vi "esp8266_test1.3.vi"() -> ()   [LabVIEW 2012]
doc: "1.2.2\n加入手动破解无线功能\n1.2.3\n由手动改为半自动破解\n1.2.4\n全自动破解与半自动破解并存模式"
uses:
  <vilib>/Instr/_visa.llb/VISA Configure Serial Port (Instr).vi
panel:
  out "String":string
  out "正常":bool
  out "透传":bool
  in  "停止":bool
  out "错误输出 2":errorcluster caption="错误输出"
  in  "清空":bool
  in  "?":enum32{"配置", "选网", "远程", "接口", "关于"}(tab)
  in  "VISA":refnum<visa-resource-name> caption="VISA资源名称"
  in  "baud rate (9600)":u32=9600
  in  "data bits (8)":u16=8 min=5 max=8 step=1
  in  "修改波特率":bool
  in  "组合框":string(combo)
  in  "模式设置":bool
  in  "模式":u32(ring) items=["无", "station模式", "AP模式", "双工模式"]
  in  "连接状态":bool
  in  "模式":bool
  in  "版本":bool
  in  "重启":bool
  in  "口令":string
  in  "name":string
  in  "连接":bool
  in  "搜索":bool
  in  "目标ID":u32(ring) items=["0", "1", "2", "3"]
  in  "响应":bool
  in  "断开":bool
  in  "发送":bool
  in  "字符串":string
  in  "关透传":bool
  in  "开透传":bool
  in  "启动":bool
  in  "本地IP":bool
  in  "MUX(1)":bool
  in  "关闭":bool
  in  "开启":bool
  in  "服务端口":string
  in  "访问":bool
  in  "端口":i32
  in  "IP":string
  in  "协议":string(combo)
  # "本软件只适用于无线\n模块的连接调试，\n  如需扩展其他功能请\n联系admin。"
  # "模块连接串口后，点击 打开"
  # "374869091"
  # "功能：\n    模块搜索附近的无线 连接到指定SSID"
  # "作者：374869091@qq.com\n版本：hello web1.2\n只适用于8266无线模块\n            \n                           2015.10"
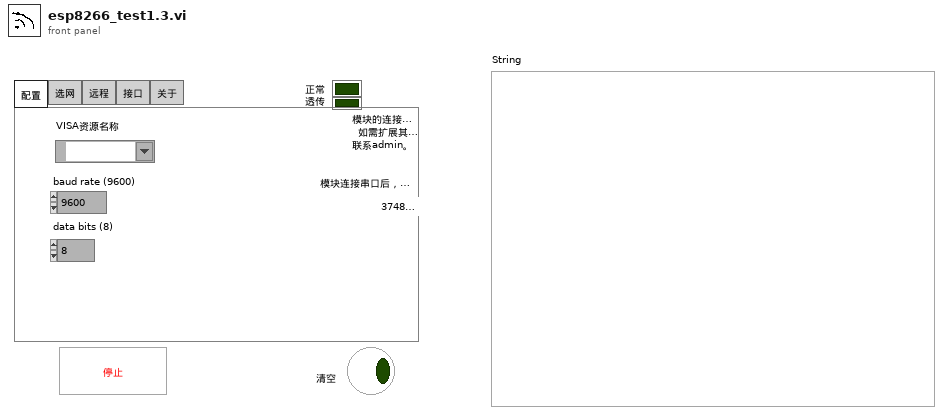
[diagram p1: front panel]
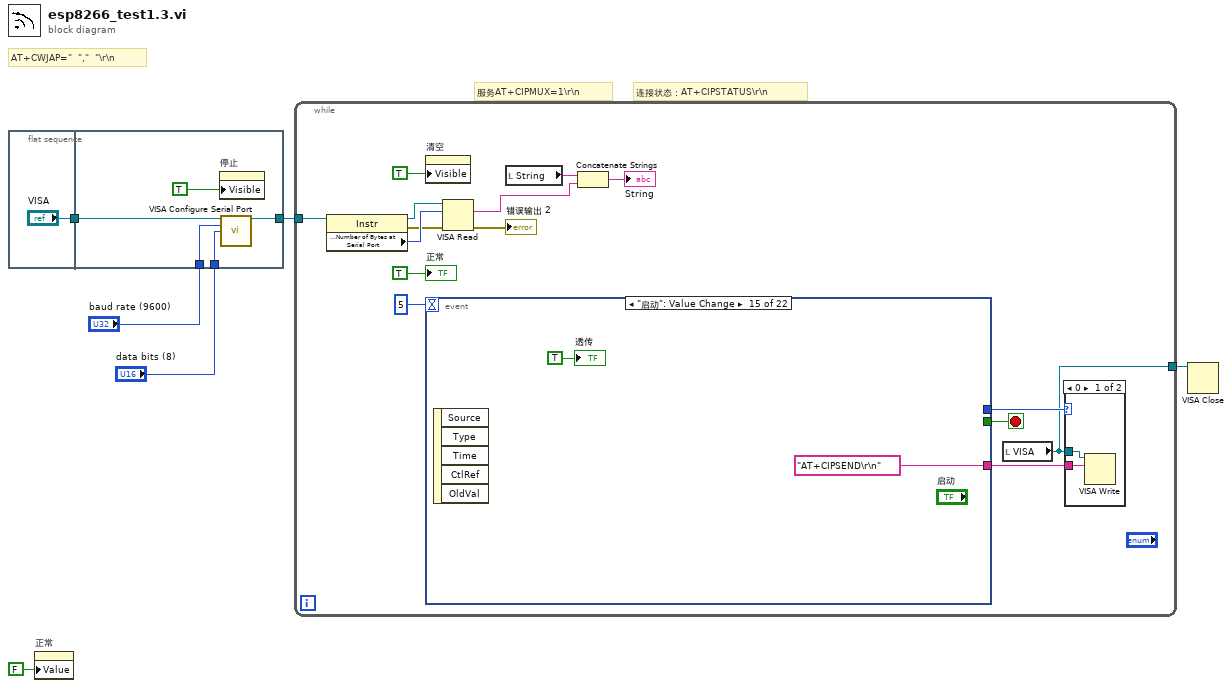
[diagram p0: block diagram]
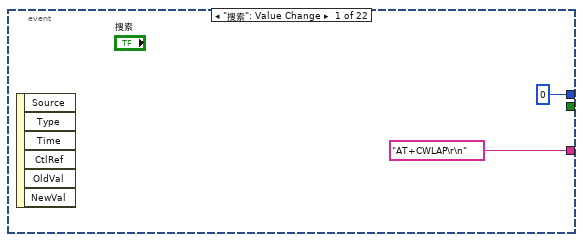
[diagram p3: hidden frame]
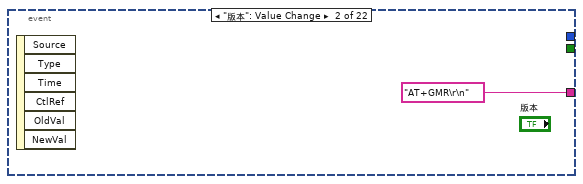
[diagram p4: hidden frame]
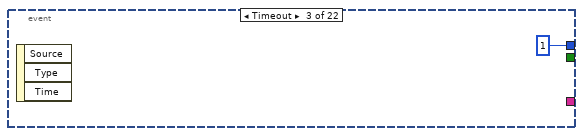
[diagram p5: hidden frame]
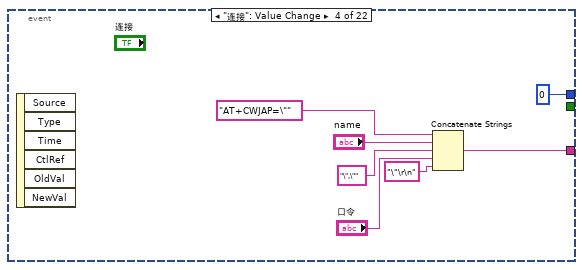
[diagram p6: hidden frame]
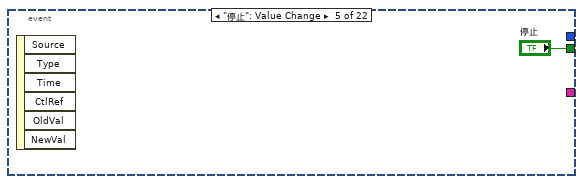
[diagram p7: hidden frame]
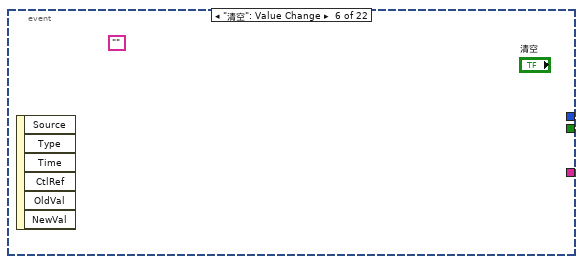
[diagram p8: hidden frame]
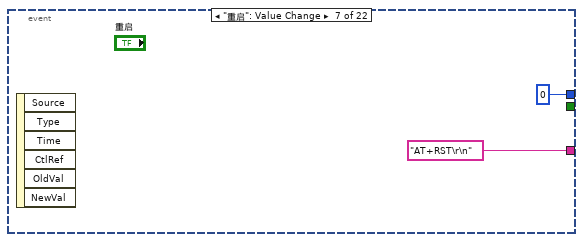
[diagram p9: hidden frame]
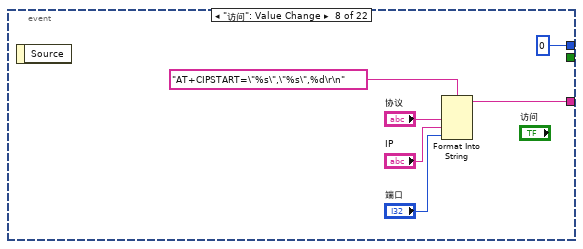
[diagram p10: hidden frame]
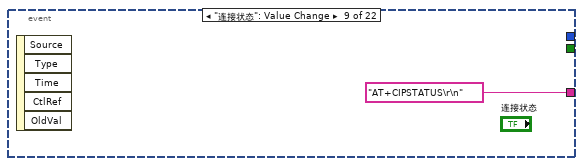
[diagram p11: hidden frame]
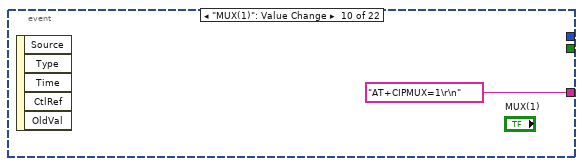
[diagram p12: hidden frame]
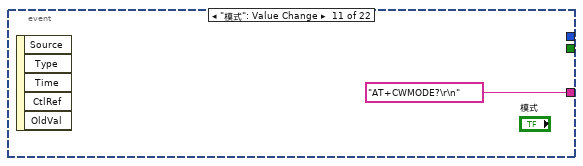
[diagram p13: hidden frame]
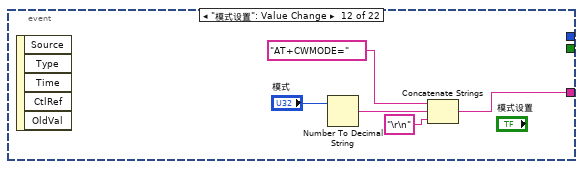
[diagram p14: hidden frame]
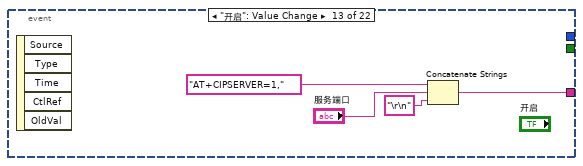
[diagram p15: hidden frame]
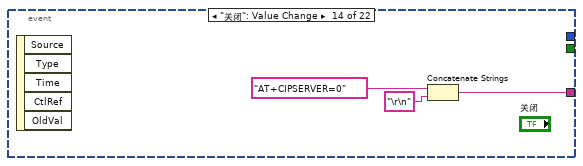
[diagram p16: hidden frame]
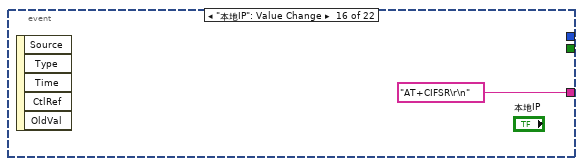
[diagram p17: hidden frame]
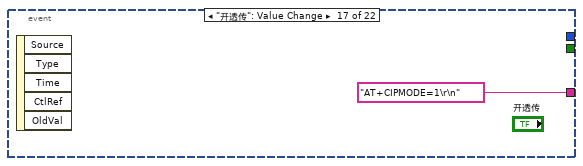
[diagram p18: hidden frame]
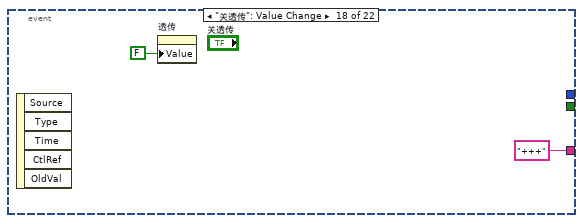
[diagram p19: hidden frame]
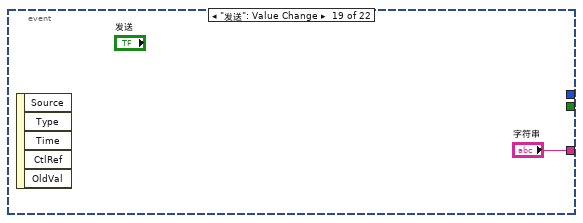
[diagram p20: hidden frame]
diagram:
  # "服务AT+CIPMUX=1\\r\\n"
  # "连接状态：AT+CIPSTATUS\\r\\n"
  # "AT+CWJAP=\"  \",\"  \"\\r\\n"
  n1 = flat-sequence {
    tunnel: ["VISA"] -> w6
    tunnel: w6 -> [w11]
    tunnel: [w10] -> w3
    tunnel: "data bits (8)" -> [w9]
    tunnel: "baud rate (9600)" -> [w8]
    frame #0 {
    }
    frame #1 {
      n2 = property on="停止" class="Bool"("Visible"=TRUE ("可见")) -> ()  [unwired: 2 in, 2 out]
      n3 = call-poly "VISA Configure Serial Port"("VISA resource name"=w11, "baud rate (9600)"=w8, "data bits (8)"=w9) -> ("VISA resource name out"=w10:refnum<visa-resource-name>)  [unwired: 11 in, 1 out]
    }
  }
  n4 = property on="正常" class="Bool (strict)"("Value"=FALSE ("正常")) -> ()  [unwired: 2 in, 2 out]
  n5 = while {
    tunnel: [w16] -> w5
    tunnel: w3 -> [w17]
    stop <- w27 stop-if-true
    n6 = property class="Instr"(reference=w17) -> (reference out=w21:refnum<visa-resource-name>, error out=w19:errorcluster, "Serial Settings:Number of Bytes at Serial Port"=w25:u32)  [unwired: 1 in]
    n7 = property on="清空" class="Bool"("Visible"=TRUE ("可见")) -> ()  [unwired: 2 in, 2 out]
    n8 = event shown="[14] \"启动\": Value Change" {
      selector: _ -> [_ _ _ _ _ _ _ _ _ _ _ _ _ _ _ _ _ _ _ _ _ _]
      dyn-events: _ -> [_ _ _ _ _ _ _ _ _ _ _ _ _ _ _ _ _ _ _ _ _ _]
      timeout: 5 -> [_ _ _ _ _ _ _ _ _ _ _ _ _ _ _ _ _ _ _ _ _ _]
      tunnel: [_ _ _ _ "停止" _ _ _ _ _ _ _ _ _ _ _ _ _ _ _ _ _] -> w27
      tunnel: ["AT+CWLAP\r\n" "AT+GMR\r\n" _ w35 _ _ "AT+RST\r\n" w47 "AT+CIPSTATUS\r\n" "AT+CIPMUX=1\r\n" "AT+CWMODE?\r\n" w53 w58 w62 "AT+CIPSEND\r\n" "AT+CIFSR\r\n" "AT+CIPMODE=1\r\n" "+++" "字符串" "AT+CIPCLOSE\r\n" w83 w84] -> w22
      tunnel: [0 _ 1 0 _ _ 0 0 _ _ _ _ _ _ _ _ _ _ _ _ _ _] -> w23
      event "搜索": Value Change {
        n9 = event-data() -> ()  [unwired: 1 in, 6 out]
      }
      event "版本": Value Change {
        n10 = event-data() -> ()  [unwired: 1 in, 6 out]
      }
      event Timeout {
        n11 = event-data() -> ()  [unwired: 1 in, 3 out]
      }
      event "连接": Value Change {
        n12 = event-data() -> ()  [unwired: 1 in, 6 out]
        n13 = Concatenate Strings("AT+CWJAP=\"", "name", "\",\"", "口令", "\"\r\n") -> (w35:string)
      }
      event "停止": Value Change {
        n14 = event-data() -> ()  [unwired: 1 in, 6 out]
      }
      event "清空": Value Change {
        (unwired) ""
        n15 = event-data() -> ()  [unwired: 1 in, 6 out]
      }
      event "重启": Value Change {
        n16 = event-data() -> ()  [unwired: 1 in, 6 out]
      }
      event "访问": Value Change {
        n17 = event-data() -> ()  [unwired: 1 in, 1 out]
        n18 = Format Into String(format string="AT+CIPSTART=\"%s\",\"%s\",%d\r\n", "协议", "IP", "端口") -> (resulting string=w47:string)  [unwired: 2 in, 1 out]
      }
      event "连接状态": Value Change {
        n19 = event-data() -> ()  [unwired: 1 in, 5 out]
      }
      event "MUX(1)": Value Change {
        n20 = event-data() -> ()  [unwired: 1 in, 5 out]
      }
      event "模式": Value Change {
        n21 = event-data() -> ()  [unwired: 1 in, 5 out]
      }
      event "模式设置": Value Change {
        n22 = event-data() -> ()  [unwired: 1 in, 5 out]
        n23 = Number To Decimal String(number="模式") -> (decimal integer string=w55:string)  [unwired: 1 in]
        n24 = Concatenate Strings("AT+CWMODE=", w55, "\r\n") -> (w53:string)
      }
      event "开启": Value Change {
        n25 = event-data() -> ()  [unwired: 1 in, 5 out]
        n26 = Concatenate Strings("AT+CIPSERVER=1,", "服务端口", "\r\n") -> (w58:string)
      }
      event "关闭": Value Change {
        n27 = event-data() -> ()  [unwired: 1 in, 5 out]
        n28 = Concatenate Strings("AT+CIPSERVER=0", "\r\n") -> (w62:string)
      }
      event "启动": Value Change {
        n29 = event-data() -> ()  [unwired: 1 in, 5 out]
        "透传" <- TRUE ("透传")
      }
      event "本地IP": Value Change {
        n30 = event-data() -> ()  [unwired: 1 in, 5 out]
      }
      event "开透传": Value Change {
        n31 = event-data() -> ()  [unwired: 1 in, 5 out]
      }
      event "关透传": Value Change {
        n32 = event-data() -> ()  [unwired: 1 in, 5 out]
        n33 = property on="透传" class="Bool (strict)"("Value"=FALSE ("透传")) -> ()  [unwired: 2 in, 2 out]
      }
      event "发送": Value Change {
        n34 = event-data() -> ()  [unwired: 1 in, 5 out]
      }
      event "断开": Value Change {
        n35 = event-data() -> ()  [unwired: 1 in, 5 out]
      }
      event "响应": Value Change {
        n36 = event-data() -> ()  [unwired: 1 in, 5 out]
        n37 = local read "字符串"() -> (w74:string)
        n38 = String Length(string=w74) -> (length=w73:i32)
        n39 = Match Pattern(string=",8\r\n", regular expression="8") -> (before substring=w77:string, after substring=w76:string)  [unwired: 1 in, 2 out]
        n40 = Number To Decimal String(number="目标ID") -> (decimal integer string=w81:string)  [unwired: 1 in]
        n41 = Number To Decimal String(number=w73) -> (decimal integer string=w75:string)  [unwired: 1 in]
        n42 = Concatenate Strings("AT+CIPSEND=", w81, w77, w75, w76) -> (w83:string)
      }
      event "修改波特率": Value Change {
        n43 = event-data() -> ()  [unwired: 1 in, 5 out]
        n44 = Concatenate Strings("AT+CIOBAUD=" ("字符串"), "组合框", "\r\n" ("字符串")) -> (w84:string)
      }
    }
    n45 = VISA Read(VISA resource name=w21, byte count=w25, error in (no error)=w19) -> (read buffer=w24:string, error out=→"错误输出 2":errorcluster)  [unwired: 2 out]
    n46 = local read "String"() -> (w15:string)
    n47 = Concatenate Strings(w15, w24) -> (→"String":string)
    n48 = local read "VISA"() -> (w16:refnum<visa-resource-name>)
    n49 = case shown="0" w23 {
      tunnel: w22 -> [w28 _]
      tunnel: w16 -> [w29 _]
      frame 0 {
        n50 = VISA Write(VISA resource name=w29, write buffer=w28) -> ()  [unwired: 1 in, 3 out]
      }
      frame 1, Default {
      }
    }
    "正常" <- TRUE ("正常")
  }
  n51 = VISA Close(VISA resource name=w5) -> ()  [unwired: 1 in, 1 out]
